vi "Initialize.vi"(8 "error in (no error)":errorcluster, 9 "Start All?":bool=TRUE, 10 "Service List":path, 11 "MicronManager in":refnum<class "MicronManager.lvclass">) -> (0 "error out":errorcluster, 2 "Services":string[](array[string]), 3 "MicronManager out":refnum<class "MicronManager.lvclass">)   [LabVIEW 2019, in "MicronManager.lvclass"]
uses:
  MicronManager.lvclass
  MicronManager.lvclass/MicronManager.ctl
  <vilib>/SLL Toolkit/SLL Table/_SubVIs/Get Column Data.vi
  <vilib>/SLL Toolkit/SLL Table/_SubVIs/Get Table Data.vi
  <vilib>/SLL Toolkit/SLL File IO/Spreadsheet/SLL Spreadsheet.lvlib
  <vilib>/SLL Toolkit/SLL Table/SLL Table.lvclass
  <vilib>/SLL Toolkit/SLL File IO/SLL File IO.lvlib
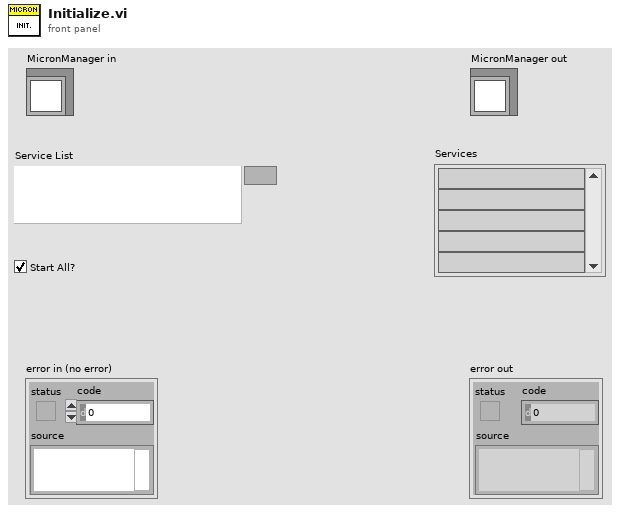
[diagram p1: front panel]
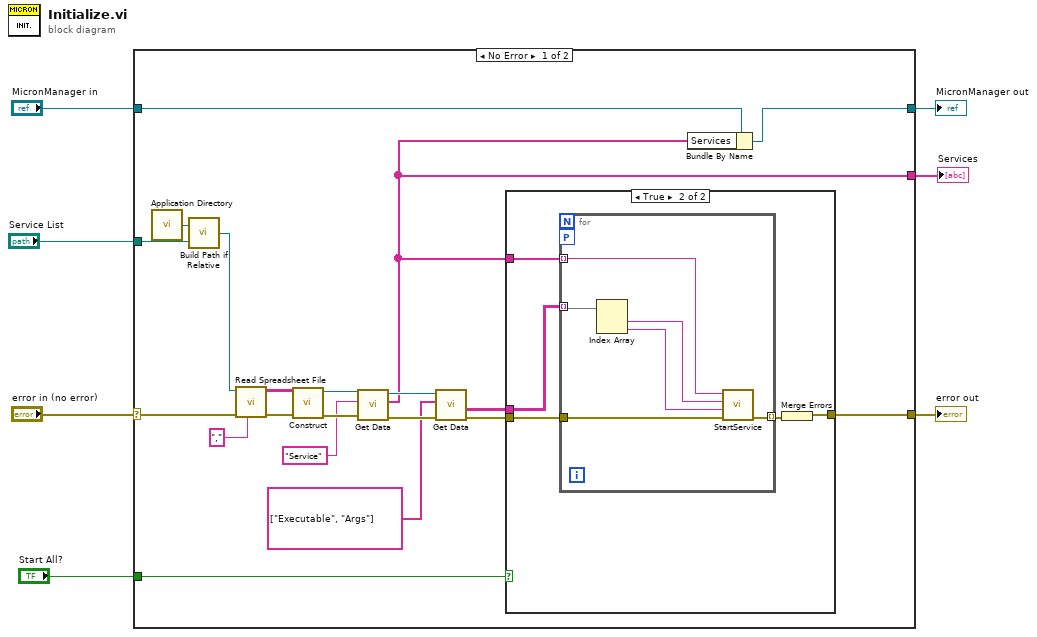
[diagram p0: block diagram]
diagram:
  n1 = case shown="No Error" "error in (no error)" {
    selector: "error in (no error)" -> [w21 w41]
    tunnel: [w12 w41] -> w6
    tunnel: [w19 w40] -> w4
    tunnel: "MicronManager in" -> [w20 w40]
    tunnel: "Service List" -> [w9 _]
    tunnel: [w13 _] -> w2
    tunnel: "Start All?" -> [w11 _]
    frame No Error {
      n2 = call <vilib>:"Application Directory.vi"() -> ("Application Directory"=w10:path)
      n3 = call <vilib>:"Build Path if Relative.vi"("Relative or Absolute Path"=w9, "Base Path"=w10) -> ("Path Out"=w8:path)
      n4 = call <vilib>:"Read Spreadsheet File.vi"("Delimiter (tab)"=",", "error in (no error)"=w21, "File Path"=w8) -> ("error out"=w26:errorcluster, "2D Array"=w25:string[][])  [unwired: 7 in]
      n5 = call <vilib>:"Construct.vi"("error in (no error)"=w26, "2D String with Headers"=w25) -> ("error out"=w24:errorcluster, "Table"=w23:refnum<class "SLL Table.lvclass">)  [unwired: 8 in]
      n6 = call-poly <vilib>:"Get Data.vi"("error in (no error)"=w24, "Header"="Service", "SLL Table in"=w23) -> ("error out"=w18:errorcluster, "Data[]"=w13:string[], "SLL Table out"=w17:refnum<class "SLL Table.lvclass">)  [unwired: 5 in, 1 out]
      n7 = call-poly <vilib>:"Get Data.vi"("error in (no error)"=w18, "Header Order[] (Optional)"=string[] ["Executable", "Args"], "SLL Table in"=w17) -> ("error out"=w14:errorcluster, "2D Data Out[][]"=w15:string[][])  [unwired: 5 in, 2 out]
      n8 = case shown="True" w11 {
        tunnel: w15 -> [_ w33]
        tunnel: w14 -> [w28 w32]
        tunnel: w13 -> [_ w30]
        tunnel: [w28 w29] -> w12
        frame False {
        }
        frame True {
          n9 = for {
            tunnel: w33 -> [w36] mode=indexing
            tunnel: w32 -> [w38]
            tunnel: [w39] -> w31 mode=indexing
            tunnel: w30 -> [w37] mode=indexing
            workers-P: _ -> [_]
            n10 = Index Array(array=w36) -> (element #1=w35:string, element #2=w34:string)  [unwired: 2 in]
            n11 = call "StartService.vi"("error in (no error)"=w38, "Args"=w34, "Executable"=w35, "Service Name"=w37) -> ("error out"=w39:errorcluster)  [unwired: 7 in]
          }
          n12 = Merge Errors(w31) -> (w29:errorcluster)
        }
      }
      n13 = Bundle By Name(cluster=w20, "Services"=w13) -> (w19:refnum<class "MicronManager.lvclass">)
    }
    frame Error {
    }
  }
  "error out" <- w6
  "MicronManager out" <- w4
  "Services" <- w2
